vi "close.vi"(8 "error in (no error)":errorcluster, 11 "RS232 in":refnum<class "RS232.lvclass">) -> (0 "error out":errorcluster, 3 "RS232 out":refnum<class "RS232.lvclass">)   [LabVIEW 2012, in "RS232.lvclass"]
uses:
  RS232.lvclass
  RS232.lvclass/RS232.ctl
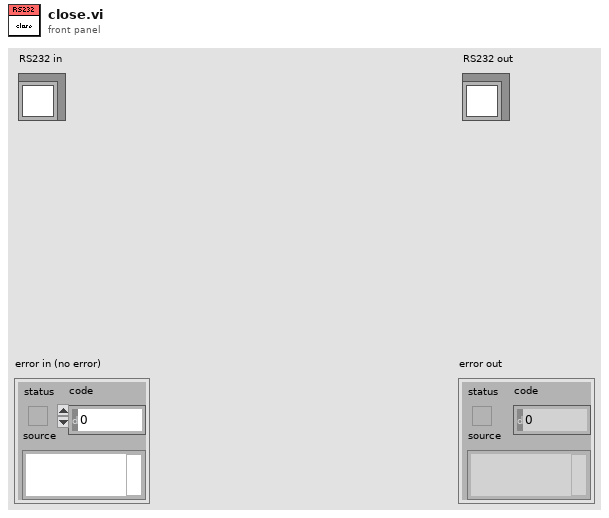
[diagram p1: front panel]
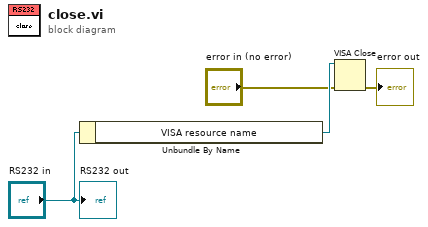
[diagram p0: block diagram]
diagram:
  n1 = Unbundle By Name("RS232 in") -> ("VISA resource name"=w3:refnum<visa-resource-name>)
  n2 = VISA Close(VISA resource name=w3, error in (no error)="error in (no error)") -> (error out=→"error out":errorcluster)
  "RS232 out" <- "RS232 in"
